vi "SyncLoop.vi"(8 "error in (no error)":errorcluster, 11 "SyncPluginBase in":refnum<class "SyncPluginBase.lvclass">) -> (0 "error out":errorcluster, 1 "Lock":bool, 2 "Time Ref Offset (ns)":dbl format="%#_12f", 3 "SyncPluginBase out":refnum<class "SyncPluginBase.lvclass">, 4 "LostLock":bool, 6 "ObtainLock":bool)   [LabVIEW 2014, in "SyncPlugins.lvlib" / "SyncPluginBase.lvclass"]
uses:
  SyncPluginBase.lvclass
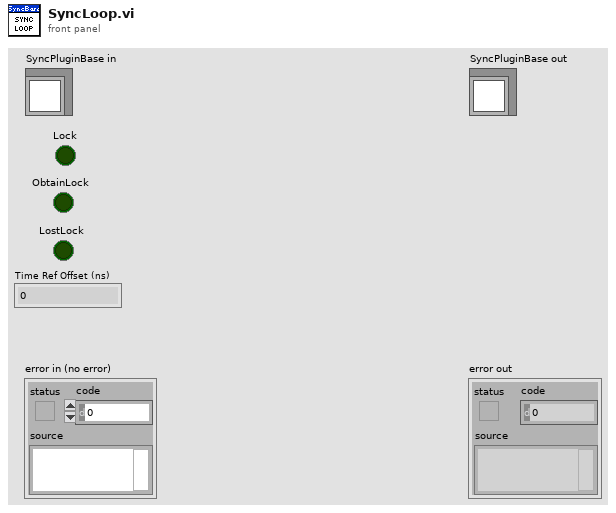
[diagram p1: front panel]
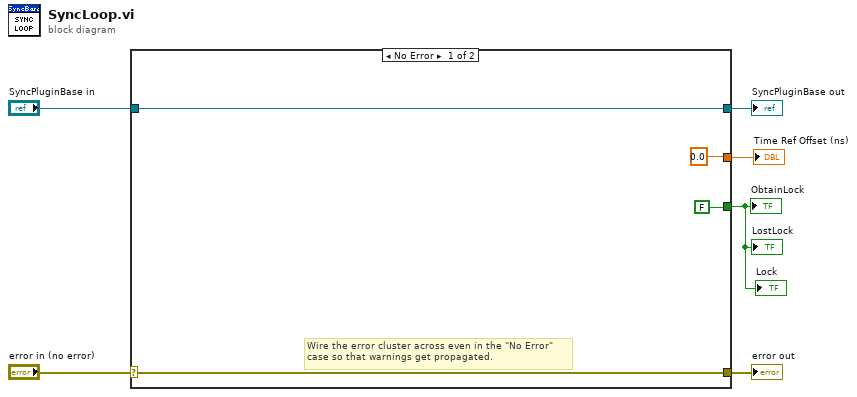
[diagram p0: block diagram]
diagram:
  n1 = case shown="No Error" "error in (no error)" {
    selector: "error in (no error)" -> [w9 w12]
    tunnel: [w9 w12] -> w5
    tunnel: [w10 w11] -> w3
    tunnel: "SyncPluginBase in" -> [w10 w11]
    tunnel: [FALSE _] -> w1
    tunnel: [0.0 _] -> w2
    frame No Error {
      # "Wire the error cluster across even in the \"No Error\"\ncase so that warnings get propagated."
    }
    frame Error {
    }
  }
  "error out" <- w5
  "SyncPluginBase out" <- w3
  "ObtainLock" <- w1
  "LostLock" <- w1
  "Time Ref Offset (ns)" <- w2
  "Lock" <- w1
